vi "ZLIB Open Zip Stream__ogtk.vi"(4 "error in (no error)":errorcluster, 6 "append (create new)":T1, 7 "archive stream":string) -> (0 "error out":errorcluster, 2 "globalComment":string, 3 "zip Refnum":T2)   [LabVIEW 2011]
doc: "Opens a zip session."
uses:
  <userlib>/_OpenG.lib/lvzip/lvzip.llb/ZLIB Zip Handle__ogtk.ctl
  <userlib>/_OpenG.lib/lvzip/lvzip.llb/ZLIB Open ZIP Mode__ogtk.ctl
  <userlib>/_OpenG.lib/lvzip/lvzlib.dll
panel:
  # "Please visit http://www.OpenG.org to learn about the\nOpen Source LabVIEW software movement.\n\nNOTICE -- YOU MUST LEAVE THIS NOTICE IN PLACE.  PER THE TERMS OF THE LICENSE BELOW, YOU MAY SUBLICENSE THIS SOFTWARE \nIN ANY WAY THAT DOES NOT CONFLICT WITH THIS LICENSE.\n\n### BSD License (http://www.opensource.org/licenses/bsd-license.php) Begin ###\n \nCopyright (C) 2002-2007 Rolf Kalbermatter rolf.kalbermatter@citeng.com\nCopyright (C) 2002 Jim Kring jim@jimkring.com\n\nAll rights reserved.\n\nRedistribution and use in source and binary forms, with or without modification, are permitted provided that the following conditions are met:\n\n    * Redistributions of source code must retain the above copyright notice, this list of conditions and the following disclaimer.\n    * Redistributions in binary form must reproduce the above copyright notice, this list of conditions and the following disclaimer in the \n       documentation and/or other materials provided with the distribution.\n    * Neither the name of SciWare, James Kring, Inc., nor the names of its contributors may be used to endorse or promote products derived \n       from this software without specific prior written permission.\n\nTHIS SOFTWARE IS PROVIDED BY THE COPYRIGHT HOLDERS AND CONTRIBUTORS \"AS IS\" AND ANY EXPRESS OR IMPLIED WARRANTIES, \nINCLUDING, BUT NOT LIMITED TO, THE IMPLIED WARRANTIES OF MERCHANTABILITY AND FITNESS FOR A PARTICULAR PURPOSE ARE \nDISCLAIMED. IN NO EVENT SHALL THE COPYRIGHT OWNER OR CONTRIBUTORS BE LIABLE FOR ANY DIRECT, INDIRECT, INCIDENTAL,\n SPECIAL, EXEMPLARY, OR CONSEQUENTIAL DAMAGES (INCLUDING, BUT NOT LIMITED TO, PROCUREMENT OF SUBSTITUTE GOODS OR \nSERVICES; LOSS OF USE, DATA, OR PROFITS; OR BUSINESS INTERRUPTION) HOWEVER CAUSED AND ON ANY THEORY OF LIABILITY, \nWHETHER IN CONTRACT, STRICT LIABILITY, OR TORT (INCLUDING NEGLIGENCE OR OTHERWISE) ARISING IN ANY WAY OUT OF THE USE \nOF THIS SOFTWARE, EVEN IF ADVISED OF THE POSSIBILITY OF SUCH DAMAGE.\n\n### BSD License End ###"
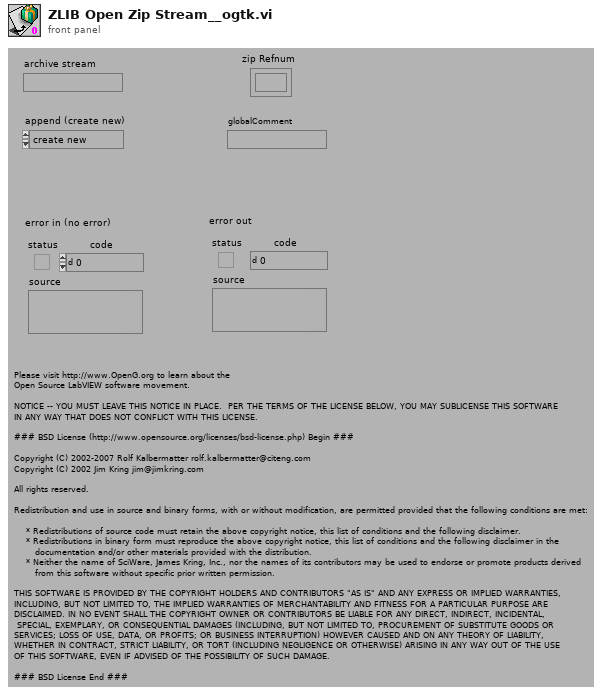
[diagram p1: front panel]
types:
  T1 = typedef "ZLIB Open ZIP Mode__ogtk.ctl" = enum16{"create new", "append to end", "append to archive"}
  T2 = typedef "ZLIB Zip Handle__ogtk.ctl" = refnum<k1>
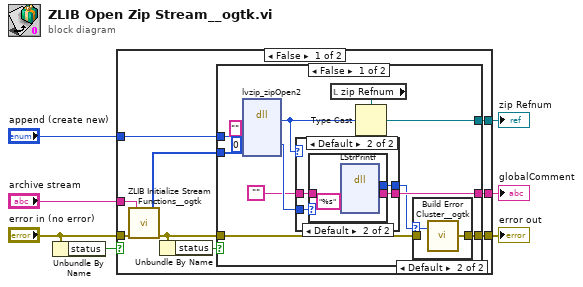
[diagram p0: block diagram]
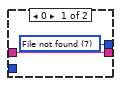
[diagram p3: hidden frame]
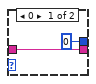
[diagram p4: hidden frame]
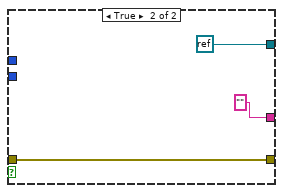
[diagram p5: hidden frame]
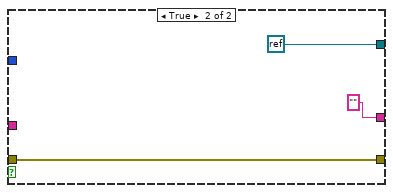
[diagram p6: hidden frame]
diagram:
  n1 = Unbundle By Name("error in (no error)") -> ("status"=w3:bool)
  n2 = case shown="False" w3 {
    tunnel: "archive stream" -> [w9 _]
    tunnel: [w16 refnum<k0> refnum] -> w6
    tunnel: "error in (no error)" -> [w8 w50]
    tunnel: [w15 w50] -> w5
    tunnel: "append (create new)" -> [w14 _]
    tunnel: [w10 "" ("dest")] -> w1
    frame False {
      n3 = call <userlib>:"ZLIB Initialize Stream Functions__ogtk.vi"("error in (no error)"=w8, "stream"=w9) -> ("error out"=w12:errorcluster, "fileFuncs"=w13:u8[])  [unwired: 4 in]
      n4 = Unbundle By Name(w12) -> ("status"=w11:bool)
      n5 = case shown="False" w11 {
        tunnel: [w28 refnum<k0> refnum] -> w16
        tunnel: [w21 w47] -> w15
        tunnel: w14 -> [w26 _]
        tunnel: w13 -> [w25 _]
        tunnel: w12 -> [w19 w47]
        tunnel: [w22 "" ("dest")] -> w10
        frame False {
          n6 = dll-call lib="C:/Development/LabVIEW 2011/user.lib/_OpenG.lib/lvzip/lvzlib.*" fn="lvzip_zipOpen2"("path"="", "append"=w26, "globalComment"=u32 0, "fileFuncs"=w25) -> (w29:u32, "globalComment"=w23:u32)  [unwired: 6 in, 2 out]
          n7 = case shown="Default" w29 {
            tunnel: w23 -> [_ w37]
            tunnel: [w33 w38] -> w22
            tunnel: [w34 w36] -> w18
            tunnel: "" -> [w33 w35]
            frame 0 {
              w34 = 7 items=["No error", "Argument error", "Memory is full", "Out of zone", "End of file", "File already open", "Generic file I/O error", "File not found", "File permission error", "Disk is full", "Duplicate path", "Too many files open", "System feature not enabled", "Resource file not found", "Cannot add resource", "Resource not found", "Image not found", "Image memory error", "Pen does not exist", "Config type invalid", "Config token not found", "Config parse error", "Config memory error", "Bad external code format", "Bad external code offset", "External code not present", "Null window", "Destroy window error", "Null menu", "Print aborted", "Bad print record", "Print driver error", "Windows error during printing", "Memory error during printing", "Print dialog error", "Generic print error", "Invalid device refnum", "Device not found", "Device parameter error", "Device unit error", "Cannot open device", "Device call aborted", "Generic error", "Cancelled by user", "Object ID too low", "Object ID too high", "Object not in heap", "Unknown heap", "Unknown object (invalid DefProc)", "Unknown object (DefProc not in table)", "Message out of range", "Invalid (null) method", "Unknown message", "Manager call not supported", "Bad address", "Network operation in progress", "Network operation timed out", "Connection is busy", "Network attribute not supported", "Network error", "Address in use", "System out of memory", "Connection aborted", "Connection refused", "Not connected", "Already connected", "Connection closed", "Initialization error (interapplication manager)", "Bad occurrence", "Wait on unbound occurrence handler", "Occurrence queue overflow", "Datalog type conflict", "Unused", "Unrecognized type (interapplication manager)", "Memory corrupt", "Failed to make temporary DLL", "Old CIN version", "Drag socket not found", "Failed to load drop-object", "Failed to register OLE object", "Failed to release OLE object", "Format specifier type mismatch", "Unknown format specifier", "Too few format specifiers", "Too many format specifiers", "Scan failed", "Newer CIN version", "Error converting to variant", "Runtime menu error", "Password tampered", "Variant attribute not found", "Incompatible variant data type", "Event data is not available", "Event Store is not present", "Occurrence is not found", "Event Queue is not created", "Event info is not available", "Refnum passed is NULL", "Error retrieving Class GUID", "Error retrieving CoClass GUID", "Error retrieving TypeLib GUID.", "Bad built application magic bytes.", "Specific driver is different from the specific driver associated with the Logical Name.", "There is no session opened to the class driver.", "Max Error", "MAX - Error with config objects", "MAX - Error loading configuration", "MAX - Group not supported"]
            }
            frame Default {
              n8 = case shown="Default" w37 {
                selector: w37 -> [_ w43]
                tunnel: [w39 w45] -> w38
                tunnel: [0 w42] -> w36
                tunnel: w35 -> [w39 w41]
                frame 0 {
                }
                frame Default {
                  n9 = dll-call lib="LabVIEW" fn="LStrPrintf"("dest"=w41, "fmt"="%s", "param"=w43) -> (w42:i32, "dest"=w45:string)  [unwired: 5 in, 2 out]
                }
              }
            }
          }
          n10 = local read "zip Refnum"() -> (w27:T2)
          n11 = Type Cast(type=w27, x=w29) -> (*(type *) &x=w28:T2)
          n12 = case shown="Default" w18 {
            selector: w18 -> [_ w31]
            tunnel: [w30 w32] -> w21
            tunnel: w19 -> [w30 _]
            frame 0 {
            }
            frame Default {
              n13 = call <userlib>:"Build Error Cluster__ogtk.vi"("code"=w31) -> ("error out"=w32:errorcluster)  [unwired: 1 in]
            }
          }
        }
        frame True {
        }
      }
    }
    frame True {
    }
  }
  "error out" <- w5
  "zip Refnum" <- w6
  "globalComment" <- w1
